vi "DCPower_VoltageConfiguration.vi"(0 "IVI Refnum in":refnum<k15>, 1 "Voltage Value By Channel":dbl[](array[numeric]), 3 "Active Channels on Instrument":bool[](array[boolean]), 4 "Channel Name Array":string[](array[string]), 5 "error in (no error)":errorcluster) -> (10 "All Channel Numbers Array":string[](array[string]), 12 "Active Channel Numbers Array":string[](array[string]), 13 "Active Channel Voltage Array":dbl[](array[numeric]), 14 "IVI Refnum out":refnum<k15>, 15 "Active Channel Names Array":string[](array[string]), 17 "Total Voltage Indicator Array":dbl[](array[numeric]), 18 "Active Channels Indicator Array":bool[](array[boolean]), 19 "error out":errorcluster)   [LabVIEW 2019]
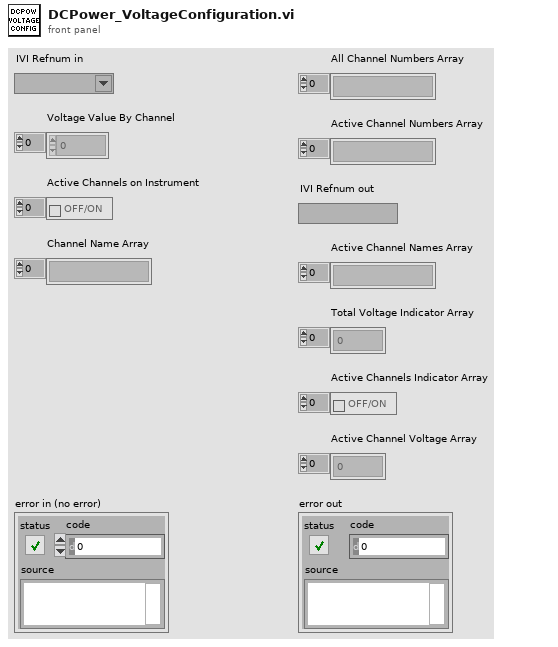
[diagram p1: front panel]
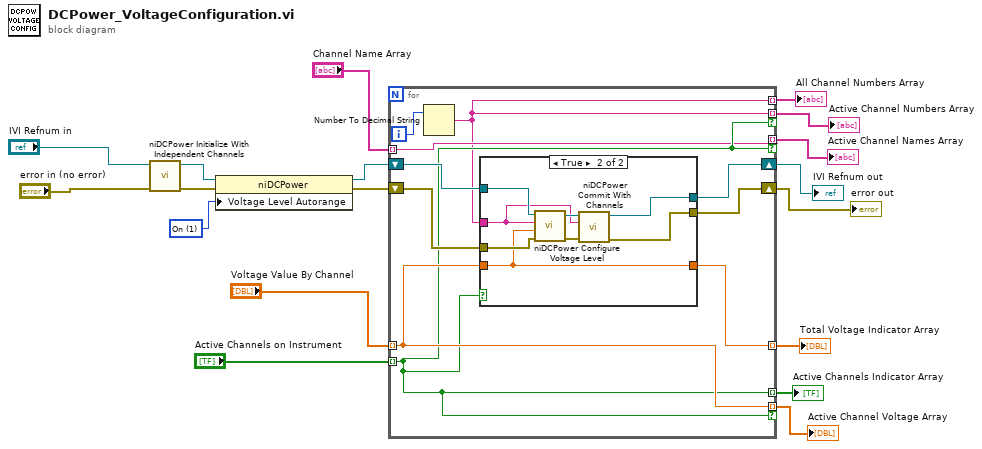
[diagram p0: block diagram]
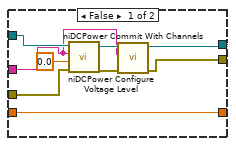
[diagram p2: hidden frame]
diagram:
  w5 = 1 items=["Off", "On"] ("Source:DC Voltage:Voltage Level Autorange")
  n1 = call <instrlib>:"niDCPower Initialize With Independent Channels.vi"("error in (no error)"="error in (no error)", "resource name"="IVI Refnum in") -> ("error out"=w3:errorcluster, "instrument handle out"=w4:refnum<k15>)  [unwired: 8 in]
  n2 = property class="niDCPower"(reference=w4, error in=w3, "Voltage Level Autorange"=w5) -> (reference out=w2:refnum<k15>, error out=w1:errorcluster)
  n3 = for {
    tunnel: "Active Channels on Instrument" -> [w24] mode=indexing
    shift-right: [w19] -> w6
    shift-left: w1 -> [w26]
    tunnel: "Voltage Value By Channel" -> [w25] mode=indexing
    tunnel: [w24] -> w17 mode=indexing
    tunnel: [w21] -> w14 mode=indexing
    tunnel: [w21] -> w8 mode=indexing if=w24
    tunnel: [w22] -> w15 mode=indexing if=w24
    tunnel: [w25] -> w18 mode=indexing if=w24
    tunnel: [w23] -> w16 mode=indexing
    tunnel: "Channel Name Array" -> [w22] mode=indexing
    shift-right: [w20] -> w7
    shift-left: w2 -> [w27]
    i -> [w28]
    n4 = Number To Decimal String(number=w28) -> (decimal integer string=w21:string)  [unwired: 1 in]
    n5 = case shown="True" w24 {
      tunnel: w27 -> [w35 w44]
      tunnel: w21 -> [w32 w42]
      tunnel: w26 -> [w34 w41]
      tunnel: [w29 w38] -> w19
      tunnel: [w30 w39] -> w20
      tunnel: w25 -> [w31 w40]
      tunnel: [w31 w40] -> w23
      frame False {
        n6 = call <instrlib>:"niDCPower Configure Voltage Level.vi"("error in (no error)"=w34, "voltage level"=0.0, "channel name"=w32, "instrument handle"=w35) -> ("error out"=w37:errorcluster, "instrument handle out"=w33:refnum<k15>)  [unwired: 6 in]
        n7 = call <instrlib>:"niDCPower Commit With Channels.vi"("error in (no error)"=w37, "channel name"=w32, "instrument handle"=w33) -> ("error out"=w29:errorcluster, "instrument handle out"=w30:refnum<k15>)  [unwired: 7 in]
      }
      frame True {
        n8 = call <instrlib>:"niDCPower Configure Voltage Level.vi"("error in (no error)"=w41, "voltage level"=w40, "channel name"=w42, "instrument handle"=w44) -> ("error out"=w45:errorcluster, "instrument handle out"=w43:refnum<k15>)  [unwired: 6 in]
        n9 = call <instrlib>:"niDCPower Commit With Channels.vi"("error in (no error)"=w45, "channel name"=w42, "instrument handle"=w43) -> ("error out"=w38:errorcluster, "instrument handle out"=w39:refnum<k15>)  [unwired: 7 in]
      }
    }
  }
  "Active Channel Voltage Array" <- w18
  "Active Channels Indicator Array" <- w17
  "Total Voltage Indicator Array" <- w16
  "error out" <- w6
  "IVI Refnum out" <- w7
  "Active Channel Names Array" <- w15
  "Active Channel Numbers Array" <- w8
  "All Channel Numbers Array" <- w14
